vi "DAQ executor.vi"(8 "results reporter":refnum<class "results reporter.lvclass">, 9 "execution system":T1=enum."standard", 10 "thread pool":refnum<class "thread pool.lvclass">, 11 "task":refnum<class "task.lvclass">) -> ()   [LabVIEW 2014, in "thread pool.lvclass"]
uses:
  thread pool.lvclass
  task/task.lvclass
  results reporter/results reporter.lvclass
  execution system.ctl
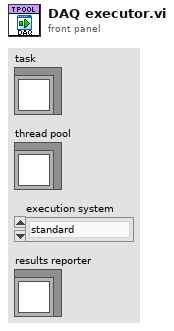
[diagram p1: front panel]
types:
  T1 = typedef "thread pool.lvclass/execution system.ctl" = enum32{"user interface", "standard", "instrument i/o", "data acquisition", "other 1", "other 2"}
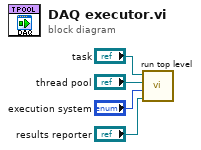
[diagram p0: block diagram]
diagram:
  n1 = call "run top level.vi"("results reporter"="results reporter", "execution system"="execution system", "thread pool"="thread pool", "task"="task") -> ()  [unwired: 8 in]
